vi "Comments com.vi"(1 "command text in":string[](array[string]), 2 "option":T1) -> (0 "Command text out":string[][](array[string]))   [LabVIEW 2025]
doc: "Author: Scott Hannahs <sth@magnet.fsu.edu>\n\nThis software is licensed for use under the “MIT License\"\nCopyright (c) 2025 Scott Hannahs, sth@sth@magnet.sthnet.net\n\nPermission is hereby granted, free of charge, to any person obtaining a copy of this software and associated documentation files (the \"Software\"), to deal in the Software without restriction, including without limitation the rights to use, copy, modify, merge, publish, distribute, sublicense, and/or sell copies of the Software, and to permit persons to whom the Software is furnished to do so, subject to the following conditions: The above copyright notice and this permission notice shall be included in all copies or substantial portions of the Software.\n\nTHE SOFTWARE IS PROVIDED \"AS IS\", WITHOUT WARRANTY OF ANY KIND, EXPRESS OR IMPLIED, INCLUDING BUT NOT LIMITED TO THE WARRANTIES OF MERCHANTABILITY, FITNESS FOR A PARTICULAR PURPOSE AND NONINFRINGEMENT. IN NO EVENT SHALL THE AUTHORS OR COPYRIGHT HOLDERS BE LIABLE FOR ANY CLAIM, DAMAGES OR OTHER LIABILITY, WHETHER IN AN ACTION OF CONTRACT, TORT OR OTHERWISE, ARISING FROM, OUT OF OR IN CONNECTION WITH THE SOFTWARE OR THE USE OR OTHER DEALINGS IN THE SOFTWARE."
uses:
  Ctl/option.ctl
panel:
  in  "comment string":string
  in  "enter":bool
  in  "cancel":bool
  # "Insert Comments"
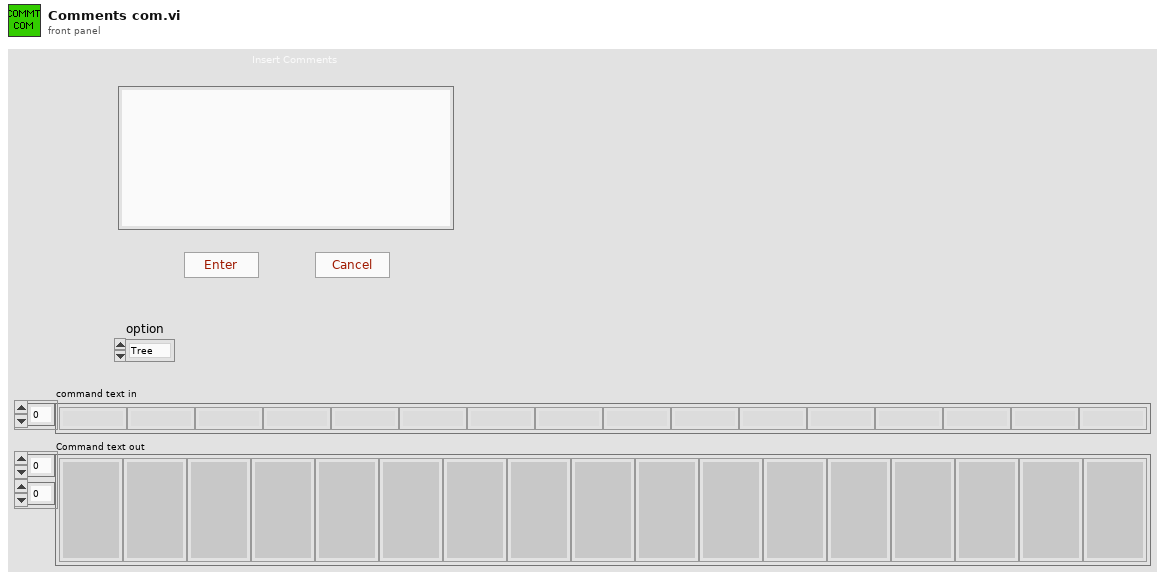
[diagram p1: front panel]
types:
  T1 = typedef "option.ctl" = enum16{"Tree", "List"}
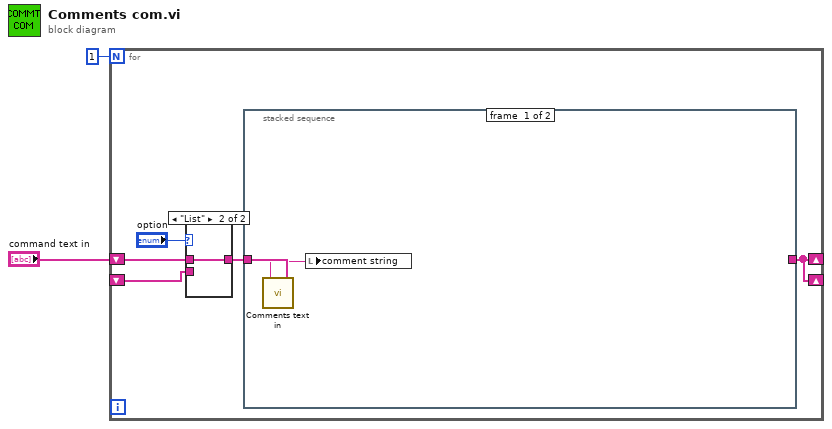
[diagram p0: block diagram]
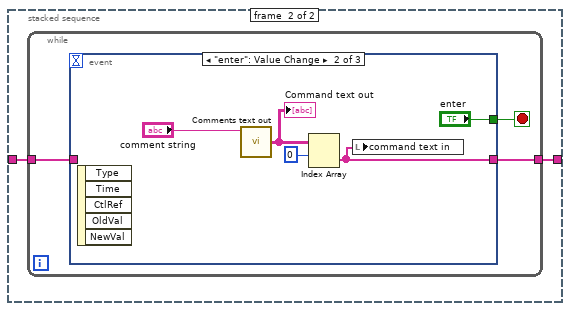
[diagram p3: hidden frame]
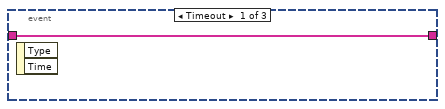
[diagram p4: hidden frame]
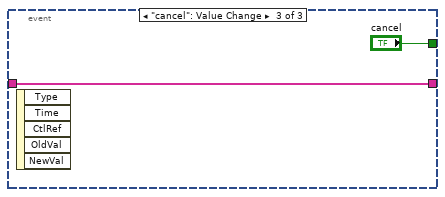
[diagram p5: hidden frame]
diagram:
  n1 = for {
    N: 1 -> [_]
    shift-right: [w3] -> _
    shift-left: _ -> [w4]
    shift-right: [w3] -> _
    shift-left: "command text in" -> [w6]
    n2 = case shown="\"List\"" "option" {
      tunnel: [w8 w9] -> w5
      tunnel: w4 -> [w8 _]
      tunnel: w6 -> [_ w9]
      frame "Tree", Default {
      }
      frame "List" {
      }
    }
    n3 = stacked-sequence {
      tunnel: [_ w13] -> w3
      tunnel: w5 -> [w11 w12]
      frame #0 {
        n4 = call "Comments text in.vi"("command text in"=w11) -> ("commet string"=w10:string)
        n5 = local write "comment string"(w10) -> ()
      }
      frame #1 {
        n6 = while {
          tunnel: [w15] -> w13
          tunnel: w12 -> [w14]
          stop <- w16 stop-if-true
          n7 = event shown="[1] \"enter\": Value Change" {
            selector: _ -> [_ _ _]
            dyn-events: _ -> [_ _ _]
            timeout: _ -> [_ _ _]
            tunnel: [_ "enter" "cancel"] -> w16
            tunnel: [w17 w19 w23] -> w15
            tunnel: w14 -> [w17 _ w23]
            event Timeout {
              n8 = event-data() -> ()  [unwired: 1 in, 2 out]
            }
            event "enter": Value Change {
              n9 = event-data() -> ()  [unwired: 1 in, 5 out]
              n10 = call "Comments text out.vi"("comment string"="comment string") -> ("Command text"=w21:string[][])  [unwired: 3 in]
              "Command text out" <- w21
              n11 = Index Array(array=w21, index (row)=0) -> (element=w19:string[])  [unwired: 1 in]
              n12 = local write "command text in"(w19) -> ()
            }
            event "cancel": Value Change {
              n13 = event-data() -> ()  [unwired: 1 in, 5 out]
            }
          }
        }
      }
    }
  }
